vi "BBoxOneLabViewTest.vi"() -> ()   [LabVIEW 2015]
uses:
  \\mac\Home/Desktop/LabView/bbox-one-api_2015 - working/BBoxAPI.dll
  BBoxAPI.dll
panel:
  out "setBeamXY":string
  in  "Ang Y":dbl
  in  "Ang X":dbl
  out "init  result":string
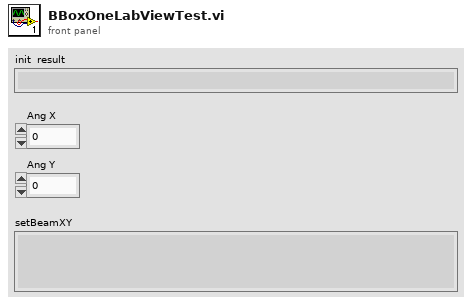
[diagram p1: front panel]
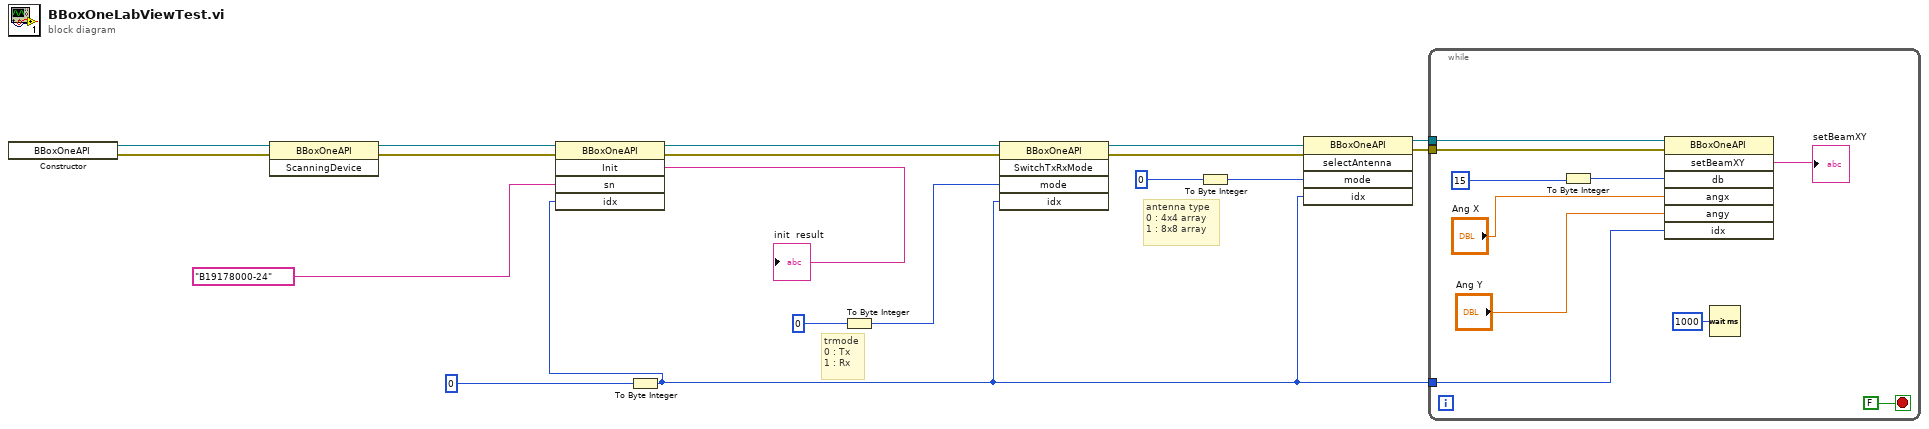
[diagram p0: block diagram]
diagram:
  # "trmode\n0 : Tx\n1 : Rx"
  # "antenna type \n0 : 4x4 array\n1 : 8x8 array"
  n1 = constructor class="BBoxOneAPI"() -> (reference out=w7:refnum<k24>, error out=w6:errorcluster)  [unwired: 3 in, 1 out]
  n2 = invoke class="BBoxOneAPI" method="ScanningDevice"(reference=w7, error in=w6) -> (reference out=w5:refnum<k24>, error out=w4:errorcluster)  [unwired: 1 in, 1 out]
  n3 = To Byte Integer(number=0) -> (8bit integer=w1:i8)
  n4 = invoke class="BBoxOneAPI" method="Init"(reference=w5, error in=w4, "sn"="B19178000-24", "idx"=w1) -> (reference out=w16:refnum<k24>, error out=w15:errorcluster, "Init"=→"init  result":string)  [unwired: 1 in, 2 out]
  n5 = To Byte Integer(number=0) -> (8bit integer=w13:i8)
  n6 = invoke class="BBoxOneAPI" method="SwitchTxRxMode"(reference=w16, error in=w15, "mode"=w13, "idx"=w1) -> (reference out=w10:refnum<k24>, error out=w9:errorcluster)  [unwired: 1 in, 3 out]
  n7 = To Byte Integer(number=0) -> (8bit integer=w11:i8)
  n8 = invoke class="BBoxOneAPI" method="selectAntenna"(reference=w10, error in=w9, "mode"=w11, "idx"=w1) -> (reference out=w3:refnum<k24>, error out=w2:errorcluster)  [unwired: 1 in, 3 out]
  n9 = while {
    tunnel: w3 -> [w28]
    tunnel: w2 -> [w27]
    tunnel: w1 -> [w22]
    stop <- FALSE stop-if-true
    n10 = To Byte Integer(number=15) -> (8bit integer=w25:i8)
    n11 = invoke class="BBoxOneAPI" method="setBeamXY"(reference=w28, error in=w27, "db"=w25, "angx"="Ang X", "angy"="Ang Y", "idx"=w22) -> ("setBeamXY"=→"setBeamXY":string)  [unwired: 1 in, 6 out]
    n12 = Wait (ms)(milliseconds to wait=u32 1000) -> ()  [unwired: 1 out]
  }
